vi "Convert temporal traces.vi"() -> ()   [LabVIEW 2012]
panel:
  out "error out":errorcluster
  in  "error in (no error)":errorcluster
  in  "Output file":path
  in  "Input file":path
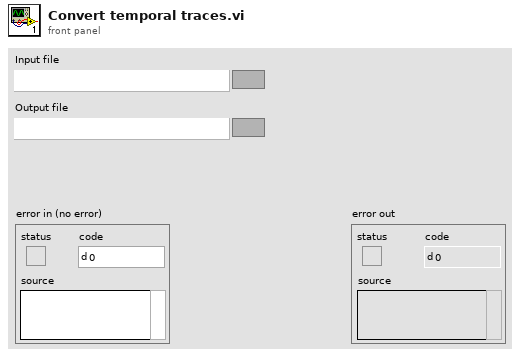
[diagram p1: front panel]
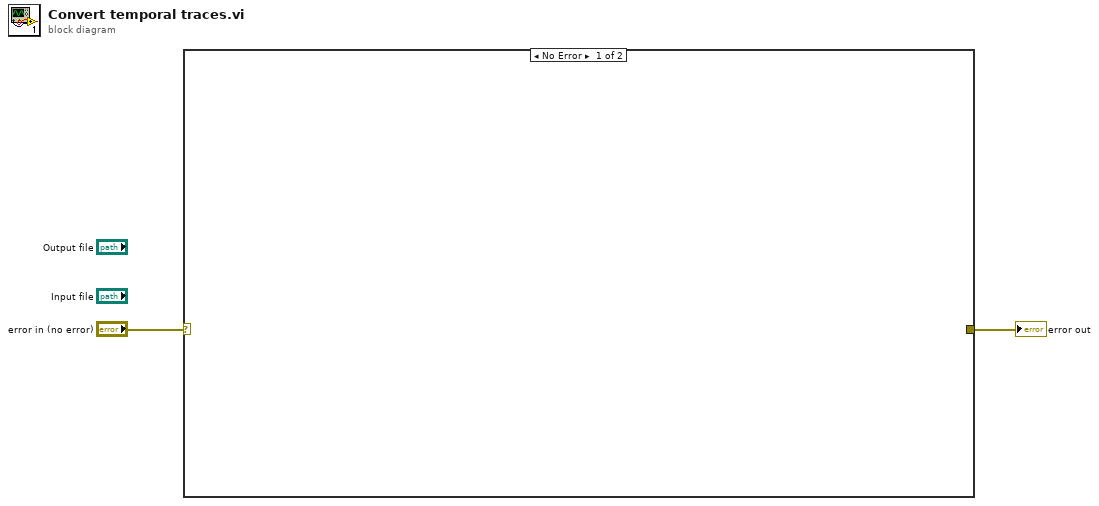
[diagram p0: block diagram]
diagram:
  n1 = case shown="No Error" "error in (no error)" {
    selector: "error in (no error)" -> [_ w3]
    tunnel: [_ w3] -> w1
    frame No Error {
    }
    frame Error {
    }
  }
  "error out" <- w1
